vi "CreatePublicEvents.vi"(8 "error in (no error)":errorcluster, 11 "0MQ_Server":refnum<class "0MQ_Server.lvclass">) -> (0 "error out":errorcluster, 3 "0MQ_Server out":refnum<class "0MQ_Server.lvclass">)   [LabVIEW 2016, in "0MQ_Server.lvclass"]
doc: "JKI State Machine Objects (SMO) 1.0.0.7\nJKI - JKI\nCopyright (c) 2016, JKI"
uses:
  0MQ_Server.lvclass
  <vilib>/addons/zeromq/poll_event_data.ctl
  0MQ_Server.lvclass/0MQ_Server.ctl
  <vilib>/JKI/JKI SMO/SMO/SMO.lvclass
  <vilib>/addons/zeromq/zeromq.lvlib
panel:
  # "For instructions on how to use the JKI State Machine Objects, examples and video tutorials, visit:\nhttp://jki.net/state-machine-objects/\n\nJKI State Machine Objects™\nhttp://jki.net/state-machine-objects/\nCopyright (C) 2005-2015, JKI <info@jki.net>\nALL RIGHTS RESERVED"
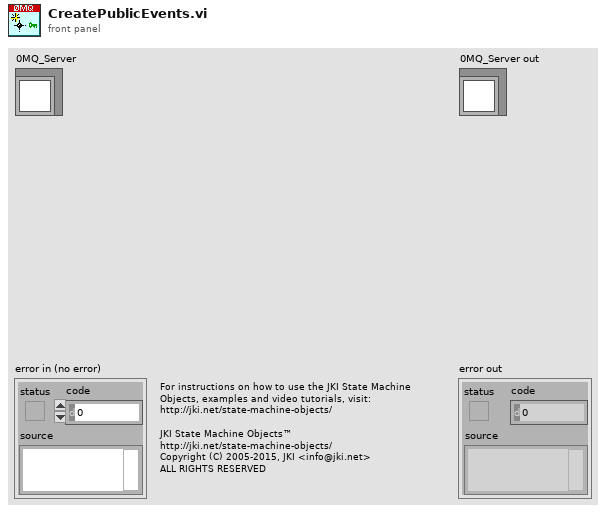
[diagram p1: front panel]
types:
  T1 = typedef "zeromq.lvlib/poll_event_data.ctl" = cluster{"identity":string, "data":string[]}
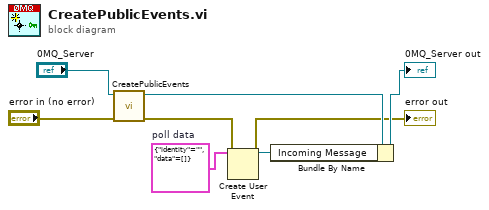
[diagram p0: block diagram]
diagram:
  w1 = T1 {"identity"="", "data"=[]}  # poll data
  n1 = call-parent "CreatePublicEvents.vi"("error in (no error)"="error in (no error)", "SMO"="0MQ_Server") -> ("error out"=w3:errorcluster, "SMO out"=w6:refnum<class "0MQ_Server.lvclass">)  [unwired: 8 in]
  n2 = Create User Event(user event datatype=w1, error in=w3) -> (user event=w4:refnum<user-event>, error out=→"error out":errorcluster)
  n3 = Bundle By Name(cluster=w6, "Incoming Message"=w4) -> (→"0MQ_Server out":refnum<class "0MQ_Server.lvclass">)
